vi "GetType.vi"(8 "error in (no error)":errorcluster, 11 "Set Output Voltage Msg":refnum<class "Set Output Voltage Msg.lvclass">) -> (0 "error out":errorcluster, 2 "Data Sample":variant, 3 "Set Output Voltage Msg":refnum<class "Set Output Voltage Msg.lvclass">)   [LabVIEW 2016, in "BNT_DAQmx.lvlib" / "Set Output Voltage Msg.lvclass"]
uses:
  Set Output Voltage Msg.lvclass
  Set Output Voltage Msg.lvclass/Set Output Voltage Msg.ctl
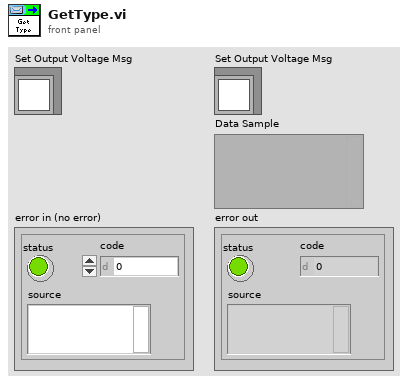
[diagram p1: front panel]
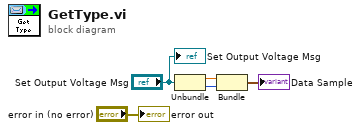
[diagram p0: block diagram]
diagram:
  n1 = Unbundle("Set Output Voltage Msg") -> (w2:dbl[unit], w1:i32)
  n2 = Bundle("Voltage"=w2, "Channel"=w1) -> (→"Data Sample":cluster{"Voltage":dbl[unit], "Channel":i32})  [unwired: 1 in]
  "error out" <- "error in (no error)"
  "Set Output Voltage Msg" <- "Set Output Voltage Msg"
